vi "Rpm of wheel  (SubVI) lab 4.vi"(9 "Diameter of wheel in inches":dbl(knob) scale=0.0..10.0) -> (3 "Velocity":dbl(knob) scale=0.0..5.0)   [LabVIEW 2016]
panel:
  out "Circumference":dbl(knob) scale=0.0..500.0
  out "Time":dbl(knob) scale=0.0..200.0
  in  "Motor's RPM":dbl(knob) scale=0.0..500.0
  out "Speed Level":dbl(slide) scale=0.0..5.0
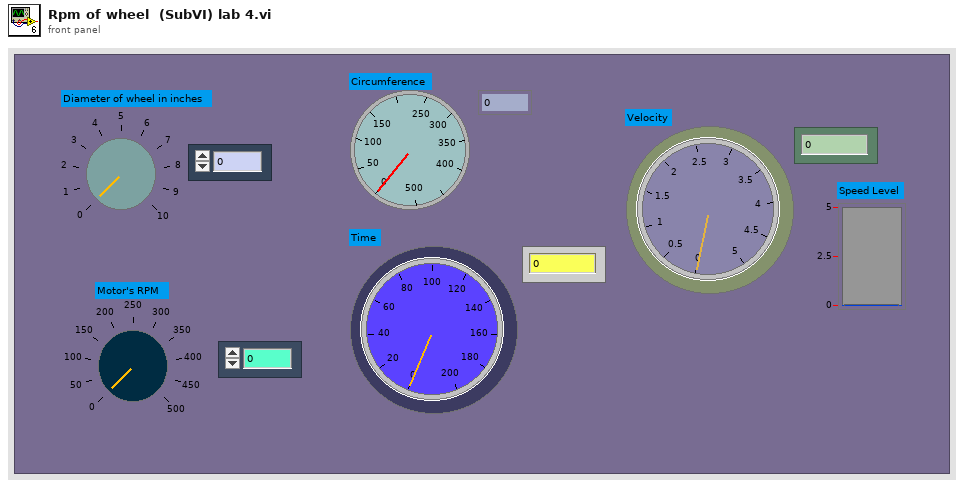
[diagram p1: front panel]
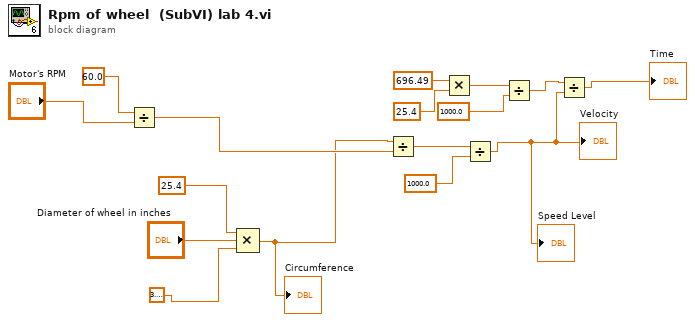
[diagram p0: block diagram]
diagram:
  n1 = Divide(x=60.0, y="Motor's RPM") -> (x/y=w11:dbl)
  n2 = Compound Arithmetic op=MULTIPLY(25.4 ("value"), "Diameter of wheel in inches", 3.141592653589793) -> (w10:dbl)
  "Circumference" <- w10
  n3 = Divide(x=w10, y=w11) -> (x/y=w9:dbl)
  n4 = Multiply(x=696.49, y=25.4) -> (x*y=w5:dbl)
  n5 = Divide(x=w9, y=1000.0) -> (x/y=w3:dbl)
  "Velocity" <- w3
  "Speed Level" <- w3
  n6 = Divide(x=w5, y=1000.0 ("x/y")) -> (x/y=w2:dbl)
  n7 = Divide(x=w2, y=w3) -> (x/y=→"Time":dbl)
